vi "JoystickSend.vi"(6 "Epsilon":dbl, 8 "error in (no error)":errorcluster, 10 "Joystick Value":dbl, 11 "Notifier Name":string="Joystick") -> (0 "error out":errorcluster)   [LabVIEW 2013]
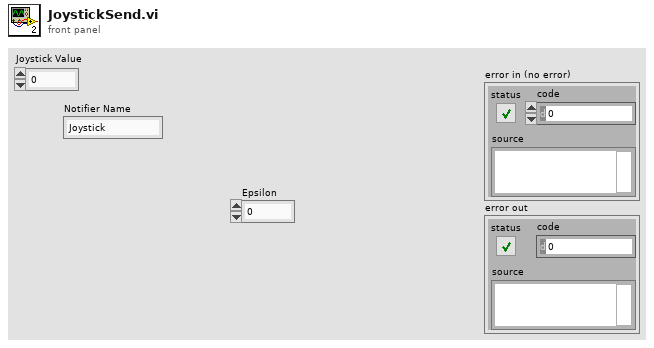
[diagram p1: front panel]
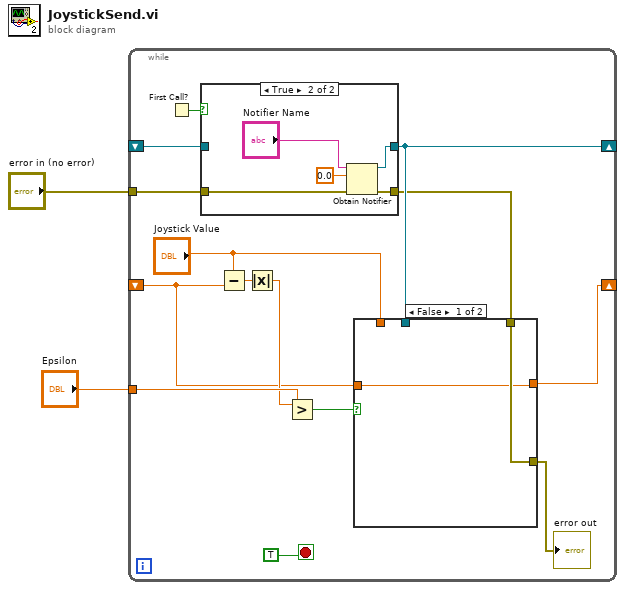
[diagram p0: block diagram]
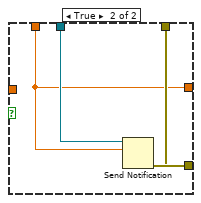
[diagram p2: hidden frame]
diagram:
  n1 = while {
    shift-right: [w10] -> _
    shift-left: _ -> [w13]
    tunnel: "error in (no error)" -> [w14]
    shift-right: [w4] -> _
    shift-left: _ -> [w3]
    tunnel: "Epsilon" -> [w12]
    stop <- TRUE stop-if-true
    n2 = First Call?() -> (First Call?: T/F=w15:bool)
    n3 = case shown="True" w15 {
      tunnel: [w24 w26] -> w10
      tunnel: w14 -> [w23 w27]
      tunnel: w13 -> [w24 _]
      tunnel: [w23 w25] -> w7
      frame False {
      }
      frame True {
        n4 = Obtain Notifier(name (unnamed)="Notifier Name", notification data type=0.0, error in (no error)=w27) -> (notifier out=w26:refnum<notifier>, error out=w25:errorcluster)  [unwired: 1 in, 1 out]
      }
    }
    n5 = Subtract(x="Joystick Value", y=w3) -> (x-y=w6:dbl)
    n6 = Absolute Value(x=w6) -> (abs(x)=w5:dbl)
    n7 = Greater?(x=w5, y=w12) -> (0:w11:bool)
    n8 = case shown="False" w11 {
      tunnel: w10 -> [_ w22]
      tunnel: "Joystick Value" -> [_ w19]
      tunnel: [w18 w21] -> w8
      tunnel: w7 -> [w18 w20]
      tunnel: [w17 w19] -> w4
      tunnel: w3 -> [w17 _]
      frame False {
      }
      frame True {
        n9 = Send Notification(notification=w19, notifier=w22, error in (no error)=w20) -> (error out=w21:errorcluster)  [unwired: 1 out]
      }
    }
    "error out" <- w8
  }
